vi "edit io channel.vi"(6 "user event":T2, 7 "Properties:instance identifier":string, 8 "error in":errorcluster, 9 "line":T1={"eip channels"=refnum, "tag name"=""}, 10 "engine configuration in":refnum<class "engine configuration.lvclass">, 11 "EthernetIP configuration in":refnum<class "EthernetIP configuration.lvclass">=refnum) -> (0 "error out":errorcluster, 2 "engine configuration out":refnum<class "engine configuration.lvclass">, 3 "EthernetIP configuration out":refnum<class "EthernetIP configuration.lvclass">)   [LabVIEW 2013, in "EIP Tag API editor node.lvclass"]
uses:
  EIP Tag API editor node.lvclass
  <vilib>/CEF_TreeControl/Controls/EventCluster.ctl
  <vilib>/CEF_TreeControl/NISE_CEF_TreeControl.lvlib
  <vilib>/NI/Module Execution Interface/Engine Configuration/engine configuration.lvclass
  <vilib>/NI/Tag Bus/tag/tag descriptor.lvclass
  <vilib>/CEF_TreeControl/Node/UserEventRef.ctl
  <vilib>/CEF_TreeControl/Node/NISE_CEF_Node.lvclass
  <vilib>/NI/TBM Modules/Ethernet IP/configuration/EthernetIP configuration.lvclass
  table line.ctl
  <vilib>/NI/TBM Modules/Ethernet IP/channel/EthernetIP Channel.lvclass
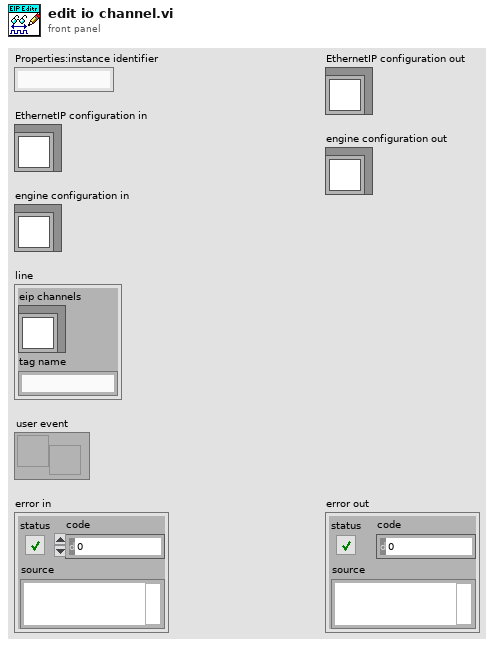
[diagram p1: front panel]
types:
  T1 = typedef "EthernetIP editor node.lvclass/table line.ctl" = cluster{"eip channels":refnum<class "EthernetIP Channel.lvclass">, "tag name":string}
  T2 = typedef "NISE_CEF_Node.lvclass/UserEventRef.ctl" = refnum<user-event>
  T3 = typedef "NISE_CEF_TreeControl.lvlib/EventCluster.ctl" = cluster{"command":string, "data":string}
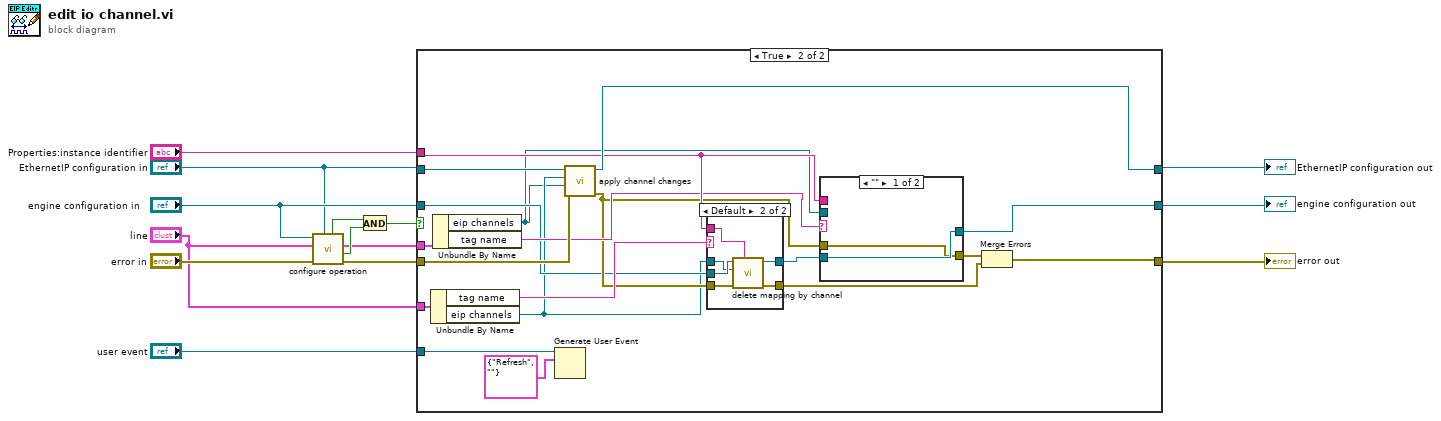
[diagram p0: block diagram]
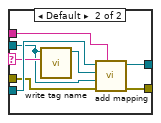
[diagram p3: hidden frame]
diagram:
  n1 = call "configure operation.vi"("EthernetIP configuration"="EthernetIP configuration in", "error in"="error in", "line item in"="line", "engine configuration in"="engine configuration in") -> ("error out"=w11:errorcluster, "success"=w14:bool, "line item out"=w3:T1, "changed"=w13:bool)  [unwired: 4 in]
  n2 = And(x=w13, y=w14) -> (x .and. y?=w10:bool)
  n3 = case shown="True" w10 {
    tunnel: [w16 w23] -> w7
    tunnel: [w17 w22] -> w8
    tunnel: "engine configuration in" -> [w17 w20]
    tunnel: w11 -> [w16 w34]
    tunnel: w3 -> [_ w31]
    tunnel: "line" -> [_ w35]
    tunnel: "EthernetIP configuration in" -> [w15 w36]
    tunnel: [w15 w30] -> w6
    tunnel: "Properties:instance identifier" -> [_ w26]
    tunnel: "user event" -> [_ w32]
    frame False {
    }
    frame True {
      n4 = Unbundle By Name(w35) -> ("tag name"=w25:string, "eip channels"=w19:refnum<class "EthernetIP Channel.lvclass">)
      n5 = Unbundle By Name(w31) -> ("eip channels"=w18:refnum<class "EthernetIP Channel.lvclass">, "tag name"=w24:string)
      n6 = Generate User Event(user event=w32, event data cluster=T3 {"command"="Refresh", "data"=""} ("event data")) -> ()  [unwired: 2 in, 2 out]
      n7 = call <vilib>:"apply channel changes.vi"("error in"=w34, 9:"TBM channel in"=w18, 10:"TBM channel in"=w19, "EthernetIP configuration in"=w36) -> ("error out"=w21:errorcluster, "EthernetIP configuration out"=w30:refnum<class "EthernetIP configuration.lvclass">)  [unwired: 6 in]
      n8 = case shown="Default" w25 {
        tunnel: w26 -> [_ w54]
        tunnel: w20 -> [w48 w53]
        tunnel: [w48 w52] -> w29
        tunnel: [w47 w51] -> w28
        tunnel: w21 -> [w47 w50]
        tunnel: w19 -> [_ w49]
        frame "" {
        }
        frame Default {
          n9 = call <vilib>:"delete mapping by channel.vi"("owner ID"=w54, "error in"=w50, "channel"=w49, "engine configuration in"=w53) -> ("error out"=w51:errorcluster, "engine configuration out"=w52:refnum<class "engine configuration.lvclass">)  [unwired: 6 in]
        }
      }
      n10 = case shown="\"\"" w24 {
        selector: w24 -> [_ w40]
        tunnel: w29 -> [w38 w46]
        tunnel: [w38 w45] -> w22
        tunnel: [w37 w44] -> w27
        tunnel: w21 -> [w37 w43]
        tunnel: w26 -> [_ w42]
        tunnel: w18 -> [_ w39]
        frame "" {
        }
        frame Default {
          n11 = call <vilib>:"write tag name.vi"("name"=w40, "system tag in"=w39) -> ("system tag out"=w41:refnum<class "tag descriptor.lvclass">)  [unwired: 8 in, 1 out]
          n12 = call <vilib>:"add mapping.vi"("owner ID"=w42, "error in"=w43, "channel"=w39, "tag descriptor"=w41, "engine configuration"=w46) -> ("error out"=w44:errorcluster, "engine configuration out"=w45:refnum<class "engine configuration.lvclass">)  [unwired: 5 in]
        }
      }
      n13 = Merge Errors(w27, w28) -> (w23:errorcluster)
    }
  }
  "engine configuration out" <- w8
  "EthernetIP configuration out" <- w6
  "error out" <- w7
